vi "External Transition.vi"(8 "error in (no error)":errorcluster, 10 "Target State":refnum<class "State Machine.lvclass">, 11 "State Machine in":refnum<class "State Machine.lvclass">) -> (0 "error out":errorcluster, 3 "State Machine out":refnum<class "State Machine.lvclass">)   [LabVIEW 2024, in "State Pattern Actor.lvlib" / "State Machine.lvlib" / "State Machine.lvclass"]
uses:
  State Machine.lvclass
  State Machine.lvclass/State Machine.ctl
  C:/Program Files (x86)/National Instruments/LabVIEW 2024/vi.lib/ActorFramework/Actor/Actor.lvclass
  C:/Users/uspoaotto/OneDrive - Oregon Tool/Desktop/working copies/stateMachineActor/src/State Pattern Actor/State Machine Actor/State Machine.lvclass
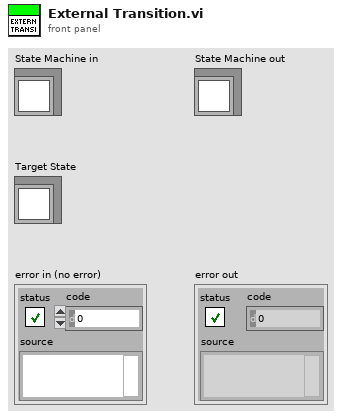
[diagram p1: front panel]
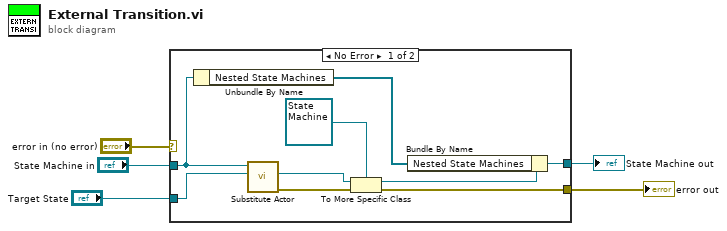
[diagram p0: block diagram]
diagram:
  n1 = case shown="No Error" "error in (no error)" {
    selector: "error in (no error)" -> [_ w16]
    tunnel: [w10 w16] -> w4
    tunnel: [w6 w15] -> w2
    tunnel: "State Machine in" -> [w9 w15]
    tunnel: "Target State" -> [w14 _]
    frame No Error {
      n2 = Unbundle By Name(w9) -> ("Nested State Machines"=w7:refnum<class "Message Enqueuer.lvclass">[])
      n3 = call-dynamic "Substitute Actor.vi"("Substitute Actor in"=w14, "Current Actor"=w9) -> ("error out"=w11:errorcluster, "Substitute Actor out"=w12:refnum<class "Actor.lvclass">)  [unwired: 8 in]
      n4 = To More Specific Class(target class=refnum<class "State Machine.lvclass"> refnum ("State Machine in 3"), reference=w12, error in=w11) -> (specific class reference=w8:refnum<class "State Machine.lvclass">, error out=w10:errorcluster)
      n5 = Bundle By Name(cluster=w8, "Nested State Machines"=w7) -> (w6:refnum<class "State Machine.lvclass">)
    }
    frame Error {
    }
  }
  "error out" <- w4
  "State Machine out" <- w2
